vi "SaveLogs.vi"(9 "Err in":string, 10 "Cmd log":T1[](array[typedef]), 11 "error log path":path) -> ()   [LabVIEW 2012]
uses:
  <userlib>/ROSforLV/ROS/Code/Console/Servers/ServerSubs/ROSLog.ctl
panel:
  out "subarray":T1[](array[typedef])
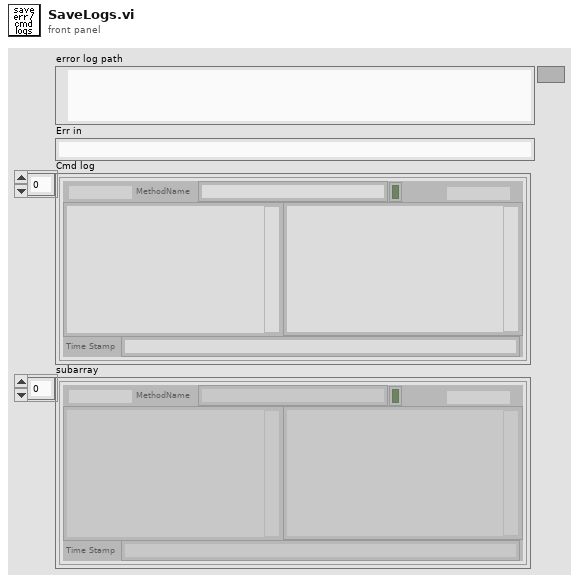
[diagram p1: front panel]
types:
  T1 = typedef "ROSLog.ctl" = cluster{"Sent":string, "Reply":string, "MethodName":string, "success":bool, "Dir1":string, "Dir2":string, "Time Stamp":string}
  T2 = cluster{"[0]":T1, "[1]":T1, "[2]":T1, "[3]":T1, "[4]":T1, "[5]":T1, "[6]":T1, "[7]":T1, "[8]":T1}
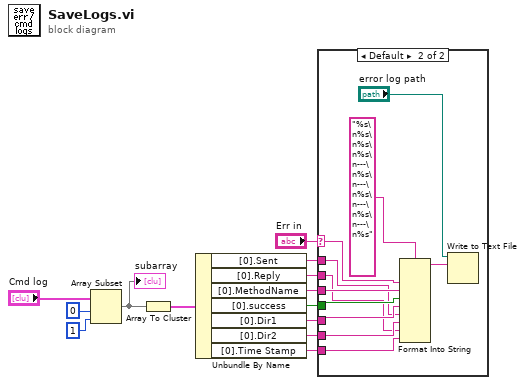
[diagram p0: block diagram]
diagram:
  n1 = Array Subset(array="Cmd log", index=0, length=1) -> (w9:T1[])
  "subarray" <- w9
  n2 = Array To Cluster(array=w9) -> (cluster=w8:T2)
  n3 = Unbundle By Name(w8) -> ("[0].Sent"=w4:string, "[0].Reply"=w2:string, "[0].MethodName"=w7:string, "[0].success"=w6:bool, "[0].Dir1"=w5:string, "[0].Dir2"=w3:string, "[0].Time Stamp"=w1:string)
  n4 = case shown="Default" "Err in" {
    selector: "Err in" -> [_ w23]
    tunnel: w7 -> [_ w22]
    tunnel: w6 -> [_ w21]
    tunnel: w5 -> [_ w20]
    tunnel: w4 -> [_ w19]
    tunnel: w3 -> [_ w18]
    tunnel: w2 -> [_ w17]
    tunnel: w1 -> [_ w16]
    frame "" {
    }
    frame Default {
      n5 = Format Into String(format string="%s\n%s\n%s\n%s\n---\n%s\n---\n%s\n---\n%s\n---\n%s", w23, w22, w21, w20, w19, w18, w17, w16) -> (resulting string=w15:string)  [unwired: 2 in, 1 out]
      n6 = Write to Text File(file (use dialog)="error log path", text=w15) -> ()  [unwired: 2 in, 3 out]
    }
  }
